vi "Create Motor State Reference.vi"(7 "state mode":T1 items=["undefined", "angle", "velocity"], 8 "error in (no error)":errorcluster) -> (0 "error out":errorcluster, 3 "motor state ref":refnum<data-value>)   [LabVIEW 2017, in "NI_Robotics_Motor Communication Ref.lvclass"]
uses:
  <vilib>/robotics/Actuation/Motor Communication Ref/NI_Robotics_Motor Communication Ref.lvclass
  <vilib>/robotics/Actuation/Motor Communication/Motor State Value.ctl
  <vilib>/robotics/Actuation/Motor Communication/Motor State Mode.ctl
  <vilib>/robotics/Actuation/Motor Communication/NI_Robotics_Motor Communication.lvclass
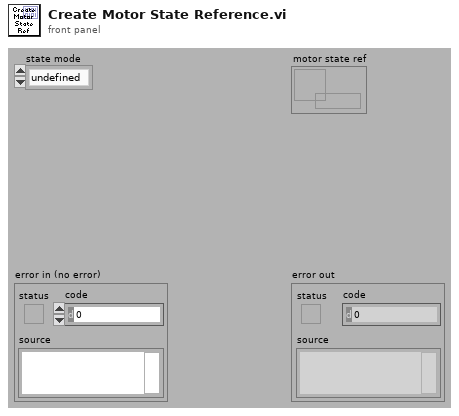
[diagram p1: front panel]
types:
  T1 = typedef "NI_Robotics_Motor Communication.lvclass/Motor State Mode.ctl" = u16
  T2 = typedef "NI_Robotics_Motor Communication.lvclass/Motor State Value.ctl" = cluster{"angle":dbl, "velocity":dbl, "state mode":T1}
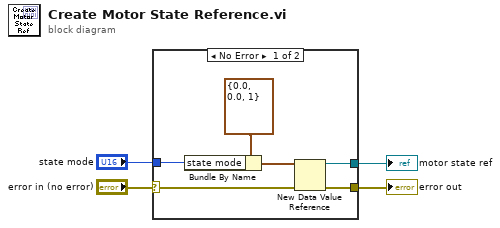
[diagram p0: block diagram]
diagram:
  n1 = case shown="No Error" "error in (no error)" {
    selector: "error in (no error)" -> [w9 w11]
    tunnel: [w10 w11] -> w4
    tunnel: [w8 _] -> w2
    tunnel: "state mode" -> [w5 _]
    frame No Error {
      n2 = Bundle By Name(cluster=T2 {"angle"=0.0, "velocity"=0.0, "state mode"=1} ("state value"), "state mode"=w5) -> (w6:T2)
      n3 = New Data Value Reference(data value=w6, error in=w9) -> (data value reference=w8:refnum<data-value>, error out=w10:errorcluster)
    }
    frame Error {
    }
  }
  "error out" <- w4
  "motor state ref" <- w2
